vi "Init.vi"(9 "Dt":dbl, 10 "Size":i32, 11 "DFT-5 in":refnum<class "DFT5.lvclass">) -> (3 "DFT-5 out":refnum<class "DFT5.lvclass">)   [LabVIEW 2014, in "Exponential Fit Library.lvlib" / "DFT5.lvclass"]
doc: "Calculate the sine and cosine of the angular frequency (wk = 2*pi*k/(N*dt)) as well as the weights used in the DFT-5 calculation. Since the average is weighted, the average of the tau's given by each of the frequency components will be sum(w_k*tau_k)/sum(w_k) where the values are summed over 1...5."
uses:
  DFT5.lvclass
  DFT5.lvclass/DFT5.ctl
  Fit Exponential.lvclass
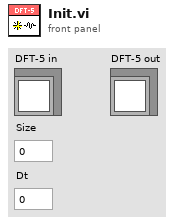
[diagram p1: front panel]
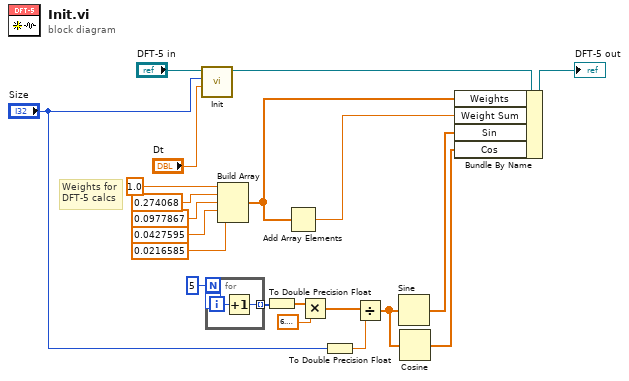
[diagram p0: block diagram]
diagram:
  # "Weights for DFT-5 calcs"
  n1 = call-parent "Init.vi"("Dt"="Dt", "Size"="Size", "Fit Exponential in"="DFT-5 in") -> ("Fit Exponential out"=w19:refnum<class "DFT5.lvclass">)  [unwired: 8 in]
  n2 = for {
    N: 5 -> [_]
    tunnel: [w22] -> w6 mode=indexing
    workers-P: _ -> [_]
    i -> [w23]
    n3 = Increment(x=w23) -> (x+1=w22:i32)
  }
  n4 = Build Array(1.0, 0.274068, 0.0977867, 0.0427595, 0.0216585) -> (w12:dbl[])
  n5 = To Double Precision Float(number=w6) -> (double precision float=w7:dbl[])
  n6 = Add Array Elements(numeric array=w12) -> (sum=w11:dbl)
  n7 = Multiply(x=w7, y=6.283185307179586) -> (x*y=w4:dbl[])
  n8 = To Double Precision Float(number="Size") -> (double precision float=w9:dbl)
  n9 = Divide(x=w4, y=w9) -> (x/y=w10:dbl[])
  n10 = Sine(x=w10) -> (sin(x)=w3:dbl[])
  n11 = Cosine(x=w10) -> (cos(x)=w2:dbl[])
  n12 = Bundle By Name(cluster=w19, "Weights"=w12, "Weight Sum"=w11, "Sin"=w3, "Cos"=w2) -> (→"DFT-5 out":refnum<class "DFT5.lvclass">)
